vi "Convert Read ERD List to Message (Rev 2 API).vi"(0 "GEA Inputs":T3 {"Destination" format="%.0x"; "Source" format="%.0x"}, 7 "ERD Read Data In":T1 {"ERD Number" format="%.0x"}, 11 "Error In":errorcluster) -> (4 "GEA Message":T4 {"Command" format="%02x"; "Destination" format="%02x"; "Source" format="%02x"}, 6 "Request ID":string, 15 "Error Out":errorcluster)   [LabVIEW 2016, in "GEA2_Toolkit.lvlib"]
doc: "This vi uses the Source / Destination from the GEA input and the ERD list to format a single GEA2 message to read the list of ERDs."
uses:
  library/GEA2_Toolkit.lvlib
  type defs/Data In.ctl
  type defs/Source_Destination.ctl
  type defs/ERD Read Data In.ctl
  type defs/Data Type.ctl
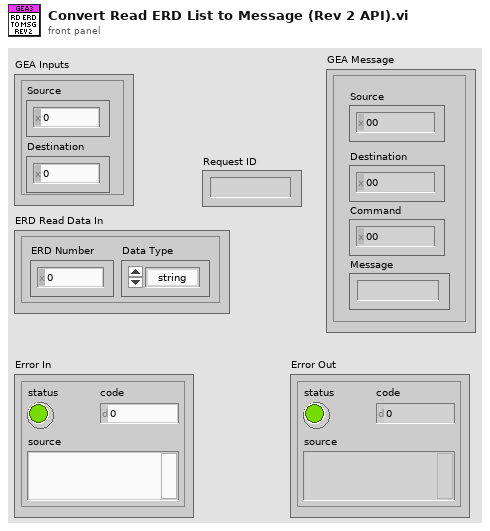
[diagram p1: front panel]
types:
  T1 = typedef "GEA2_Toolkit.lvlib/ERD Read Data In.ctl" = cluster{"ERD Number":u16, "Data Type":T2}
  T2 = typedef "GEA2_Toolkit.lvlib/Data Type.ctl" = enum16{"string", "boolean", "uint8_t", "uint16_t", "uint32_t", "uint64_t", "int8_t", "int16_t", "int32_t", "int64_t"}
  T3 = typedef "GEA2_Toolkit.lvlib/Source_Destination.ctl" = cluster{"Source":u8, "Destination":u8}
  T4 = typedef "GEA2_Toolkit.lvlib/Data In.ctl" = cluster{"Source":u8, "Destination":u8, "Command":u8, "Message":string}
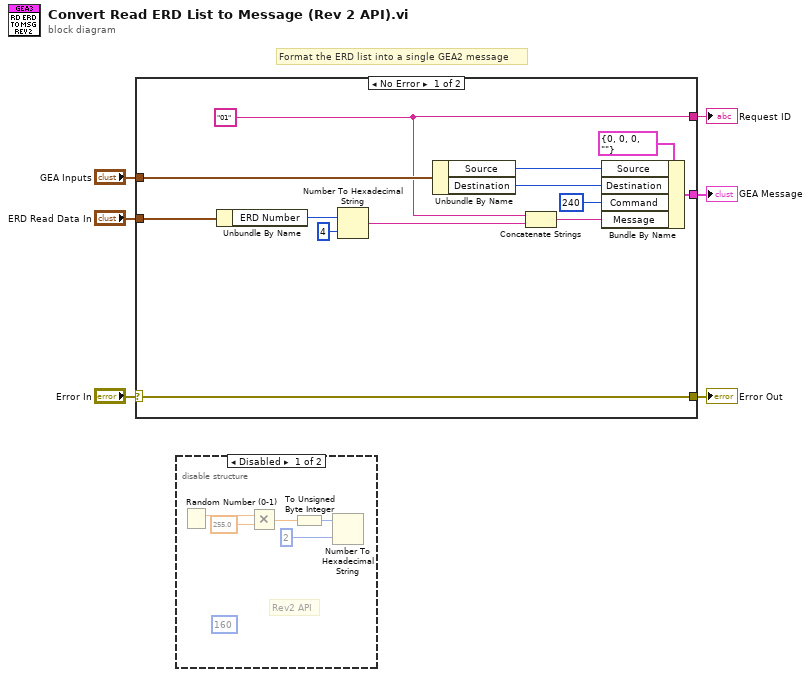
[diagram p0: block diagram]
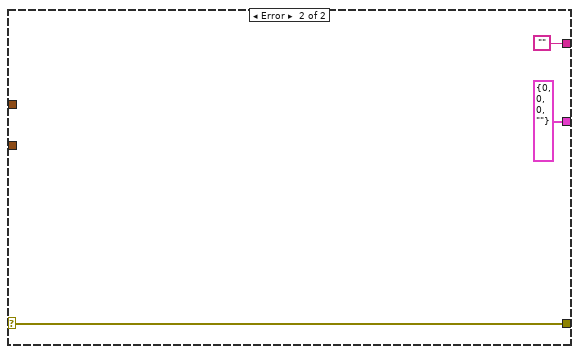
[diagram p3: hidden frame]
diagram:
  # "Format the ERD list into a single GEA2 message"
  n1 = case shown="No Error" "Error In" {
    selector: "Error In" -> [w12 w21]
    tunnel: "ERD Read Data In" -> [w8 _]
    tunnel: "GEA Inputs" -> [w18 _]
    tunnel: [w13 T4 {"Source"=0, "Destination"=0, "Command"=0, "Message"=""} ("GEA Message")] -> w5
    tunnel: [w12 w21] -> w3
    tunnel: [w7 ""] -> w2
    frame No Error {
      w7 = "01"
      n2 = Unbundle By Name(w8) -> ("ERD Number"=w10:u16)
      n3 = Number To Hexadecimal String(1:i16 4 ("width (-)"), 2:w10) -> (0:w9:string)
      n4 = Unbundle By Name(w18) -> ("Source"=w17:u8, "Destination"=w16:u8)
      n5 = Concatenate Strings(w7, w9) -> (w14:string)
      n6 = Bundle By Name(cluster=T4 {"Source"=0, "Destination"=0, "Command"=0, "Message"=""} ("GEA Message"), "Source"=w17, "Destination"=w16, "Command"=u8 240, "Message"=w14) -> (w13:T4)
    }
    frame Error {
    }
  }
  "GEA Message" <- w5
  "Error Out" <- w3
  "Request ID" <- w2
  n7 = disable-structure shown="Disabled" {
    frame Disabled {
      (unwired) u8 160 ("Command")
      # "Rev2 API"
      n8 = Random Number (0-1)() -> (number: 0 to 1=w26:dbl)
      n9 = Multiply(x=w26, y=255.0) -> (x*y=w24:dbl)
      n10 = To Unsigned Byte Integer(number=w24) -> (unsigned 8bit integer=w23:u8)
      n11 = Number To Hexadecimal String(1:i16 2 ("width (-)"), 2:w23) -> ()  [unwired: 1 out]
    }
    frame Enabled {
    }
  }
